vi "detect_preamble.vi"(8 "error in (no error)":errorcluster, 10 "Recovered Bit Sequence":i32[](array[numeric]), 11 "preamble length":i32) -> (0 "error out":errorcluster, 3 "Bit Sequence":i32[](array[numeric]))   [LabVIEW 2012]
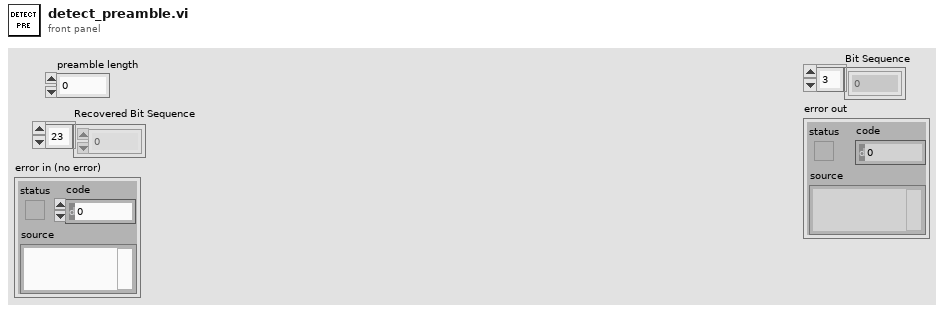
[diagram p1: front panel]
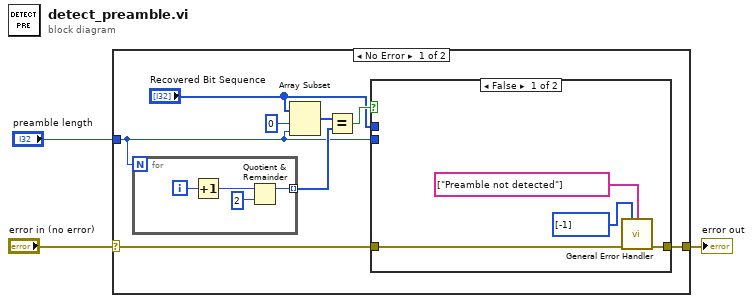
[diagram p0: block diagram]
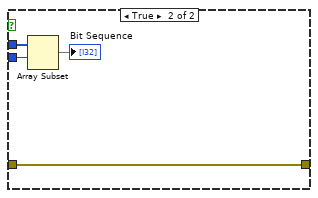
[diagram p2: hidden frame]
diagram:
  n1 = case shown="No Error" "error in (no error)" {
    selector: "error in (no error)" -> [w4 w24]
    tunnel: "preamble length" -> [w6 _]
    tunnel: [w5 w24] -> w2
    frame No Error {
      n2 = for {
        N: w6 -> [_]
        tunnel: [w12] -> w9 mode=indexing
        i -> [w15]
        n3 = Increment(x=w15) -> (x+1=w14:i32)
        n4 = Quotient & Remainder(x=w14, y=2) -> (x-y*floor(x/y)=w12:i32)  [unwired: 1 out]
      }
      n5 = Array Subset(array="Recovered Bit Sequence", index=0, length=w6) -> (w10:i32[])
      n6 = Equal?(x=w10, y=w9) -> (x = y?=w8:bool)
      n7 = case shown="False" w8 {
        tunnel: "Recovered Bit Sequence" -> [_ w23]
        tunnel: w6 -> [_ w22]
        tunnel: [w17 w20] -> w5
        tunnel: w4 -> [w16 w20]
        frame False {
          n8 = call <vilib>:"General Error Handler.vi"("[user-defined codes]"=i32[] [-1], "[user-defined descriptions]"=string[] ["Preamble not detected"], "error in (no error)"=w16) -> ("error out"=w17:errorcluster)  [unwired: 8 in, 4 out]
        }
        frame True {
          n9 = Array Subset(array=w23, index=w22) -> (→"Bit Sequence":i32[])  [unwired: 1 in]
        }
      }
    }
    frame Error {
    }
  }
  "error out" <- w2
